vi "VelocityPublisher.vi"() -> ()   [LabVIEW 2014]
uses:
  <vilib>/Tufts CEEO ROS for LabVIEW Software/ROS/Code/SubVIs/_ROSControl.ctl
  <vilib>/Tufts CEEO ROS for LabVIEW Software/ROS/Code/SubVIs/_ROSDirection.ctl
  <vilib>/Tufts CEEO ROS for LabVIEW Software/ROS/Code/Console/Servers/ServerSubs/TopicDef.ctl
panel:
  out "error out":errorcluster
  in  "End Node":bool=TRUE
  in  "Stop/Start Publishing":bool
  out "ROS Published Messages":T1={"topic port"=0, "Node"="", "topic"="", "type"="", "node port"=0, "error "={"status"=FALSE, "code"=0, "source"=""}, "Direction"=enum."Node", "Update (ms)"=1, "FIFO size"=1}
  in  "Velocity Commands":T3
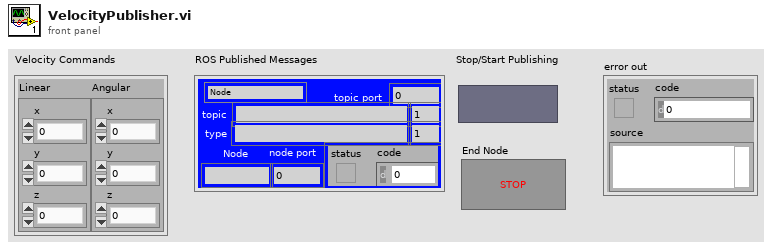
[diagram p1: front panel]
types:
  T1 = typedef "_ROSControl.ctl" = cluster{"topic port":u16, "Node":string, "topic":string, "type":string, "node port":u16, "error ":errorcluster, "Direction":T2, "Update (ms)":u16, "FIFO size":u16}
  T2 = typedef "_ROSDirection.ctl" = enum16{"Node", "Publisher", "Subscriber", "ServiceClient", "ServiceProvider"}
  T3 = cluster{"Linear":cluster{"x":dbl, "y":dbl, "z":dbl}, "Angular":cluster{"x":dbl, "y":dbl, "z":dbl}}
  T4 = typedef "TopicDef.ctl" = cluster{"Topic":string, "Type":string, "Action":T2, "Update (ms)":u16, "queue size":u16}
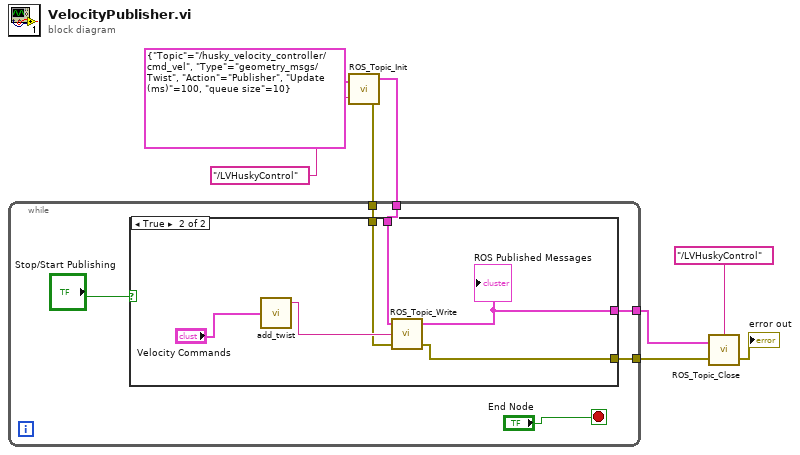
[diagram p0: block diagram]
diagram:
  n1 = call <vilib>:"ROS_Topic_Init.vi"("Definitions"=T4 {"Topic"="/husky_velocity_controller/cmd_vel", "Type"="geometry_msgs/Twist", "Action"=enum."Publisher", "Update (ms)"=100, "queue size"=10}, "node"="/LVHuskyControl" ("Node Name")) -> ("ROS out"=w7:T1, "error out"=w4:errorcluster)  [unwired: 1 in]
  n2 = while {
    tunnel: w7 -> [w14]
    tunnel: [w10] -> w6
    tunnel: [w11] -> w5
    tunnel: w4 -> [w12]
    stop <- "End Node" stop-if-true
    n3 = case shown="True" "Stop/Start Publishing" {
      tunnel: w14 -> [w15 w21]
      tunnel: w12 -> [w16 w19]
      tunnel: [w16 w18] -> w11
      tunnel: [w15 w20] -> w10
      frame False {
      }
      frame True {
        n4 = call <vilib>:"add_twist.vi"("Twist"="Velocity Commands") -> ("msg out"=w22:string)  [unwired: 4 in]
        n5 = call <vilib>:"ROS_Topic_Write.vi"("error in (no error)"=w19, "Msg in"=w22, "ROS in"=w21) -> ("error out"=w18:errorcluster, "ROS out"=w20:T1)  [unwired: 1 in]
        "ROS Published Messages" <- w20
      }
    }
  }
  n6 = call <vilib>:"ROS_Topic_Close.vi"("error in"=w5, "ROS in"=w6, "node"="/LVHuskyControl") -> ("error out"=→"error out":errorcluster)  [unwired: 1 in]
